vi "Acquire.vi"(8 "error in (no error)":errorcluster, 10 "Digital Write Status":bool[][](array[boolean]), 11 "Hardware Resources in":T1) -> (0 "error out":errorcluster, 2 "data":waveform(dbl)[](array[waveform]), 3 "Hardware Resources out":T1)   [LabVIEW 2018, in "DAQ.lvlib"]
doc: "Perform the acquisition. Replace the contents of this diagram with calls to acquisition hardware."
uses:
  DAQ/DAQ.lvlib
  Hardware Configuration.ctl
  Task Cluster.ctl
  <vilib>/DAQmx/read.llb/DAQmx Read (Analog 1D Wfm NChan NSamp).vi
  <vilib>/DAQmx/write.llb/DAQmx Write (Digital 1D Bool NChan 1Samp 1Line).vi
  <vilib>/DAQmx/miscellaneous.llb/DAQmx Fill In Error Info.vi
  <resource>/objmgr/daqmx.rc
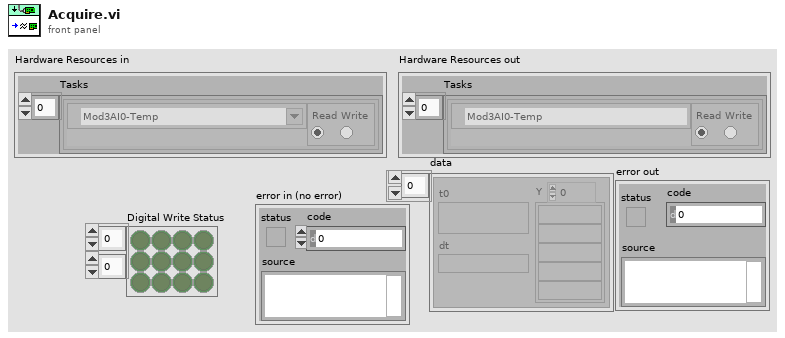
[diagram p1: front panel]
types:
  T1 = typedef "DAQ.lvlib/Hardware Configuration.ctl" = cluster{"Tasks":T2[]}
  T2 = typedef "Task Cluster.ctl" = cluster{"DAQmx Task":refnum<k21>, "Read-Write Radio":enum32{"Read", "Write"}}
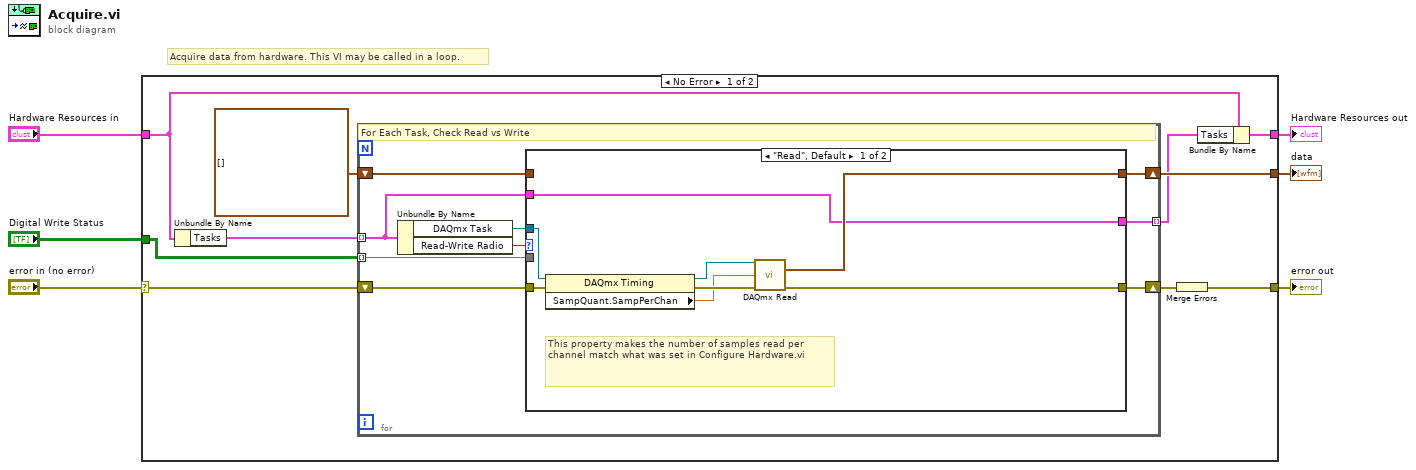
[diagram p0: block diagram]
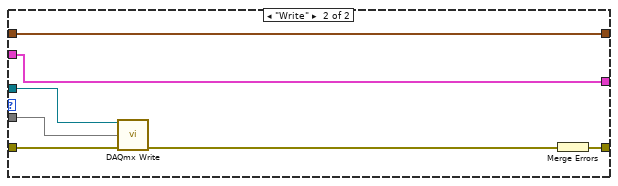
[diagram p2: hidden frame]
diagram:
  # "Acquire data from hardware. This VI may be called in a loop."
  n1 = case shown="No Error" "error in (no error)" {
    selector: "error in (no error)" -> [w13 w41]
    tunnel: [w16 w41] -> w5
    tunnel: "Hardware Resources in" -> [w9 w42]
    tunnel: [w7 w42] -> w3
    tunnel: [w11 _] -> w2
    tunnel: "Digital Write Status" -> [w12 _]
    frame No Error {
      n2 = Unbundle By Name(w9) -> ("Tasks"=w14:T2[])
      n3 = for {
        tunnel: w14 -> [w18] mode=indexing
        shift-right: [w20] -> w15
        shift-left: w13 -> [w25]
        tunnel: w12 -> [w21] mode=indexing
        shift-right: [w22] -> w11
        shift-left: waveform(dbl)[] [] ("data") -> [w19]
        tunnel: [w17] -> w8 mode=indexing
        # "For Each Task, Check Read vs Write"
        n4 = Unbundle By Name(w18) -> ("DAQmx Task"=w24:refnum<k21>, "Read-Write Radio"=w23:enum32{"Read", "Write"})
        n5 = case shown="\"Read\", Default" w23 {
          tunnel: [w26 w38] -> w20
          tunnel: w25 -> [w32 w37]
          tunnel: w24 -> [w29 w39]
          tunnel: [w28 w35] -> w22
          tunnel: w21 -> [_ w40]
          tunnel: w19 -> [_ w35]
          tunnel: w18 -> [w27 w34]
          tunnel: [w27 w34] -> w17
          frame "Read", Default {
            # "This property makes the number of samples read per channel match what was set in Configure Hardware.vi"
            n6 = property class="DAQmx Timing"(reference=w29, error in=w32) -> (reference out=w33:refnum<k21>, error out=w31:errorcluster, "SampQuant.SampPerChan"=w30:dbl)
            n7 = call-poly <vilib>:"DAQmx Read.vi"("task/channels in"=w33, "number of samples per channel"=w30, "error in"=w31) -> ("data"=w28:waveform(dbl)[], "error out"=w26:errorcluster)  [unwired: 10 in, 1 out]
          }
          frame "Write" {
            n8 = call-poly <vilib>:"DAQmx Write.vi"("task/channels in"=w39, "data"=w40, "error in"=w37) -> ("error out"=w36:errorcluster)  [unwired: 10 in, 2 out]
            n9 = Merge Errors(w36) -> (w38:errorcluster)
          }
        }
      }
      n10 = Merge Errors(w15) -> (w16:errorcluster)
      n11 = Bundle By Name(cluster=w9, "Tasks"=w8) -> (w7:T1)
    }
    frame Error {
    }
  }
  "Hardware Resources out" <- w3
  "error out" <- w5
  "data" <- w2
